vi "Dashboard Main.vi"() -> ()   [LabVIEW 2016]
uses:
  Auton Selector.ctl
  The-One-True-Robot-2017/Control Type.ctl
  <vilib>/Utility/miscctls.llb/LVRowAndColumnTypeDef.ctl
  <vilib>/event_ctls.llb/eventvkey.ctl
  <vilib>/Rock Robotics/Network Tables/NT Read Numeric Array.vi
  <vilib>/Rock Robotics/WPI/Dashboard/WPI_DashboardLogging Global.vi
  <vilib>/Rock Robotics/Network Tables/NT Write Boolean.vi
  <vilib>/Rock Robotics/Network Tables/NT Write Numeric Array.vi
  <vilib>/Rock Robotics/Network Tables/NT Write String Array.vi
panel:
  in  "Camera Settings Right":T1={"Frame Rate"=30, "Compression"=30, "Size"=1, "DB Camera Config"=FALSE} {"Frame Rate" scale=1.0..30.0; "Compression" scale=100.0..-1.0; "Size" items=["640x480", "320x240", "160x120"]}
  in  "Camera Name Right":string(combo)="No Camera Selection"
  out "Camera Info":cluster{"Mbps LED":bool, "Mbps":dbl, "fps":dbl} {"fps" format="%#.1g"; "Mbps" format="%#.1g"}
  in  "Camera Settings":T1={"Frame Rate"=30, "Compression"=30, "Size"=1, "DB Camera Config"=FALSE} {"Frame Rate" scale=1.0..30.0; "Compression" scale=100.0..-1.0; "Size" items=["640x480", "320x240", "160x120"]}
  in  "TCP":refnum<k5>
  in  "Rec Mode":enum32{"Stop", "Record", "Playback"}(radio)
  out "Robot IP":string
  out "Image Message":string="Timeout in Camera Communications"
  in  "Dashboard Tab":T2(tab)
  in  "Select Auto":T3="Select Autonomous ..."
  out "NT Connection":bool
  out "MotorChart R":cluster{"Numeric":dbl, "Numeric":dbl}(graph)
  out "MotorChart L":cluster{"Numeric":dbl, "Numeric":dbl}(graph)
  out "MotorSliders R":cluster{"MotorSlide1":dbl, "MotorSlide2":dbl} {"MotorSlide2" scale=-1.0..1.0 scale format="%#_2e"; "MotorSlide1" scale=-1.0..1.0 scale format="%#_2e"}
  out "MotorSliders L":cluster{"MotorSlide1":dbl, "MotorSlide2":dbl} {"MotorSlide2" scale=-1.0..1.0 scale format="%#_2e"; "MotorSlide1" scale=-1.0..1.0 scale format="%#_2e"}
  out "Gyro":dbl(knob) scale=0.0..360.0
  out "JS1 Z":dbl(slide) scale=-1.0..1.0 scale format="%#_2e"
  out "JS1 Graph":cluster{"X":dbl, "Y":dbl}[](graph)
  out "JS1 Buttons":T4
  out "JS2 Z":dbl(slide) scale=-1.0..1.0 scale format="%#_2e"
  out "JS2 Graph":cluster{"X":dbl, "Y":dbl}[](graph)
  out "JS2 Buttons":T4
  out "Mode":T5(ring)=enum."Auto Disabled"
  in  "Select Auto 3":T6
  out "Camera Image Right":T7(plugin-control)
  in  "DB/String 9":string
  in  "DB/String 8":string
  in  "DB/String 7":string
  in  "DB/String 6":string
  in  "DB/String 5":string
  in  "DB/String 4":string
  in  "DB/String 3":string
  in  "DB/String 2":string
  in  "DB/String 1":string
  in  "DB/String 0":string
  in  "DB/Slider 0":dbl(slide) scale=0.0..5.0
  in  "DB/Slider 1":dbl(slide) scale=0.0..5.0
  in  "DB/Slider 2":dbl(slide) scale=0.0..5.0
  in  "DB/Slider 3":dbl(slide) scale=0.0..5.0
  out "DB/LED 3":bool
  out "DB/LED 2":bool
  in  "DB/Button 3":bool
  in  "DB/Button 2":bool
  in  "DB/Button 1":bool
  in  "DB/Button 0":bool
  out "DB/LED 0":bool
  out "DB/LED 1":bool
  in  "Nintendo Camera Switch":bool
  in  "Distance":dbl
  in  "Right":dbl
  in  "Left":dbl
  in  "Toggle LED":bool
  in  "Test Slider":dbl(slide) scale=0.0..100.0 scale format="%#_3g"
  in  "On/Off":bool caption="Solenoid"
  in  "Test Name":u16(ring) items=["Select the test to run..."]
  in  "Test Tree":string(tree)
  in  "Motor":cluster{"Value":dbl, "Enable":bool} {"Value" scale=-1.0..1.0 scale format="%#_3g"}
  out "Progress":T8 {"Test Progress" scale=0.0..100.0}
  in  "Rev/Fwd":cluster{"Forward":bool, "Reverse":bool}
  in  "Test Ring":u16(ring) items=["Monochrome", "Color"]
  out "Cmd Status":string
  in  "Execute Command":bool
  in  "Command Params":string[][](table)
  in  "Command Selection":i32(listbox)
  in  "CheckList":i32(listbox)
  out "Tree":string(tree)
  out "Camera Image":T7(plugin-control)
  out "Background":bool
  in  "Camera Name":string(combo)="No Camera Selection"
  # "HW"
  # "HW"
  # "Joysticks"
  # "Drive Motors"
  # "Front"
  # "Right"
  # "Left"
  # "Back"
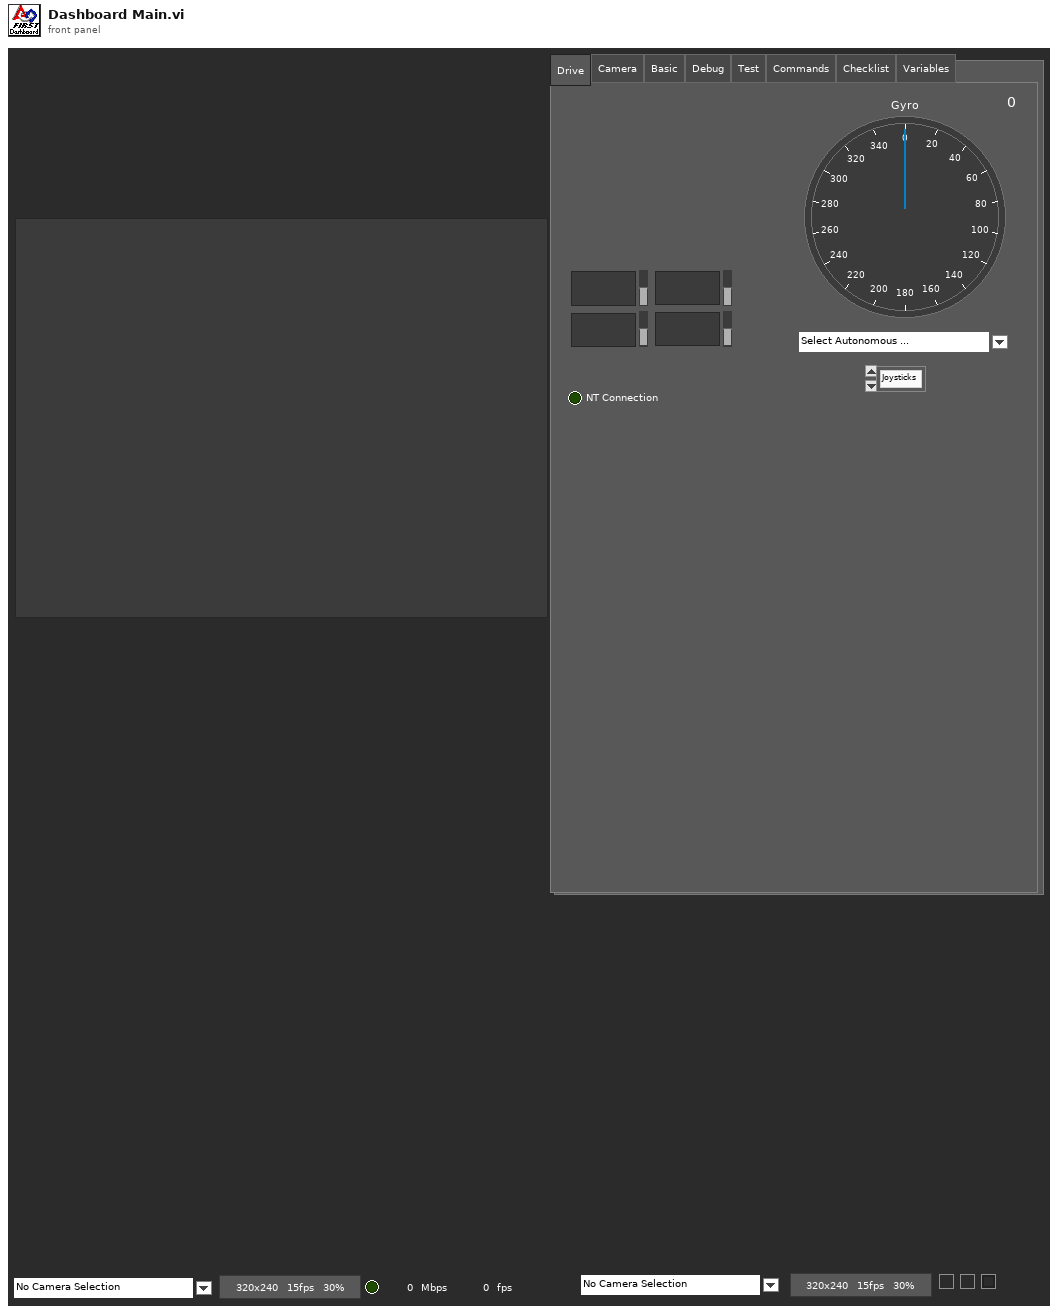
[diagram p1: front panel]
types:
  T1 = cluster{"Frame Rate":i32, "Compression":i32, "Size":u16, "DB Camera Config":bool}
  T2 = enum32{"Drive", "Camera", "Basic", "Debug", "Test", "Commands", "Checklist", "Variables"}
  T3 = typedef "Auton Selector.ctl" = string
  T4 = cluster{bool, bool, bool, bool, bool, bool, bool, bool, bool, bool, bool, bool}
  T5 = enum8{"Tele-Op Disabled", "Tele-Op Enabled", "Auto Disabled", "Auto Enabled", "Test Disabled", "Test Enabled", "Disconnected", "No Code", "E-Stop"}
  T6 = typedef "Control Type.ctl" = enum16{"Joysticks", "Xbox", "DancingRevolution"}
  T7 = typedef "IMAQ Image.ctl" = refnum<image>
  T8 = cluster{"Test Progress":u8, "Test Progress Text":string}
  T9 = typedef "Image Type" = u32
  T10 = cluster{"IDs":cluster{"RPC field ID":u16, "Unique ID":u16}, "String":string}
  T11 = enum32{"Drive", "Basic", "Debug", "Test", "Checklist", "Variables"}
  T12 = cluster{"Error Strings":string, "Disable Counts":cluster{u16, u16}, "Rail Faults":cluster{u16, u16, u16}, "Robot IP":string, "DB Mode":u8, "Event Info":cluster{"Name":string, "Type":u8, "Number":u16, "Replay":u8}}
  T13 = cluster{"Storage":cluster{"Disk Free":u64, "RAM Block":u32, "RAM free":u32}, "CPU Utilization":cluster{"CPU % ISR":sgl, "CPU % Time Crit":sgl, "CPU % Timed Str":sgl, "CPU % High":sgl, "CPU % Above":sgl, "CPU % Normal":sgl, "CPU % Low":sgl}, "CAN":cluster{"% Bus Utilization":sgl, "Bus Off Cnt":u32, "TX_FIFO Full Cnt":u32, "Receive Error Cnt":u8, "Transmit Error Cnt":u8}, "HID":cluster{"HID Outputs":u32, "Rumble Low":u16, "Rumble High":u16}[]}
  T14 = cluster{"Status bits":cluster{"Test Mode":bool, "Autonomous":bool, "Enabled":bool, "Code Start":bool, "Brownout":bool, "Reserved 2":bool, "Reserved 3":bool, "E-Stop":bool}, "Code Trace":cluster{"Disabled":bool, "TeleOp":bool, "Auto":bool, "Test":bool}, "Controller Type":enum16{"unknown", "cRIO", "roboRio"}, "Code?":enum16{"unknown", "noCode", "code"}, "Battery V":dbl}
  T15 = cluster{"Control Bits":cluster{"TestMode":bool, "Autonomous":bool, "Enabled":bool, "FMS Present":bool, bool, bool, bool, "E-Stop":bool}, "Team Station ":u8, "Countdown":sgl, "Joystick Values":cluster{"Axes":dbl[], "Buttons":bool[], "POVs":i16[]}[]}
  T16 = cluster{"Axes":dbl[], "Buttons":bool[], "POVs":i16[]}[]
  T17 = cluster{"Axes":dbl[], "Buttons":bool[], "POVs":i16[]}
  T18 = cluster{"Buttons[0]":bool, "Buttons[1]":bool, "Buttons[2]":bool, "Buttons[3]":bool, "Buttons[4]":bool, "Buttons[5]":bool, "Buttons[6]":bool, "Buttons[7]":bool, "Buttons[8]":bool, "Buttons[9]":bool, "Buttons[10]":bool, "Buttons[11]":bool}
  T19 = cluster{"Camera Image":refnum<vi>, "Dashboard Tab":refnum<vi>, "Background":refnum<vi>, "Rec Mode":refnum<vi>, "Test Slider":refnum<vi>, "On/Off ":refnum<vi>, "Test Ring":refnum<vi>, "Rev/Fwd":refnum<vi>, "Test Name":refnum<vi>, "Motor":refnum<vi>, "Progress":refnum<vi>, "CheckList":refnum<vi>, "Tree":refnum<vi>, "Test Tree":refnum<vi>, "Command Params":refnum<vi>, "Command Selection":refnum<vi>, "Execute Command":refnum<vi>, "Cmd Status":refnum<vi>, "Camera Settings":refnum<vi>, "Camera Name":refnum<vi>, "Camera Info":refnum<vi>, "Camera Settings Right":refnum<vi>, "Camera Name Right":refnum<vi>, "Camera Image Right":refnum<vi>}
  T20 = cluster{"Operation":enum16{"Update", "Clear"}, "Color Box":u32}[]
  T21 = typedef "eventvkey.ctl" = enum16{"ASCII", "Enter", "Return", "Shift", "Ctrl", "Alt", "Cmd", "Opt", "Caps", "NumLock", "Clear", "Break", "Up", "Down", "Left", "Right", "Insert", "Delete", "Home", "End", "PageUp", "PageDown", "Escape", "Help", "Pause", "ScrollLock", "F1", "F2", "F3", "F4", "F5", "F6", "F7", "F8", "F9", "F10", "F11", "F12", "F13", "F14", "F15", "F16", "F17", "F18", "F19", "F20", "F21", "F22", "F23", "F24", "Play", "VolumeUp", "VolumeDown", "Mute", "Two Byte Char"}
  T22 = cluster{"Image Size":bool, "Image Type":bool, "Pixel Value":bool, "ROI Information":bool, "Zoom Factor":bool}
  T23 = cluster{"Operation":enum16{"Update", "Clear"}, "Color Box":u32}
  T24 = typedef "LVRowAndColumnTypeDef.ctl" = cluster{"Row":i32, "Column":i32}
  T25 = cluster{"Shift":bool, "Ctrl":bool, "Alt":bool, "Cmd":bool, "Opt":bool}
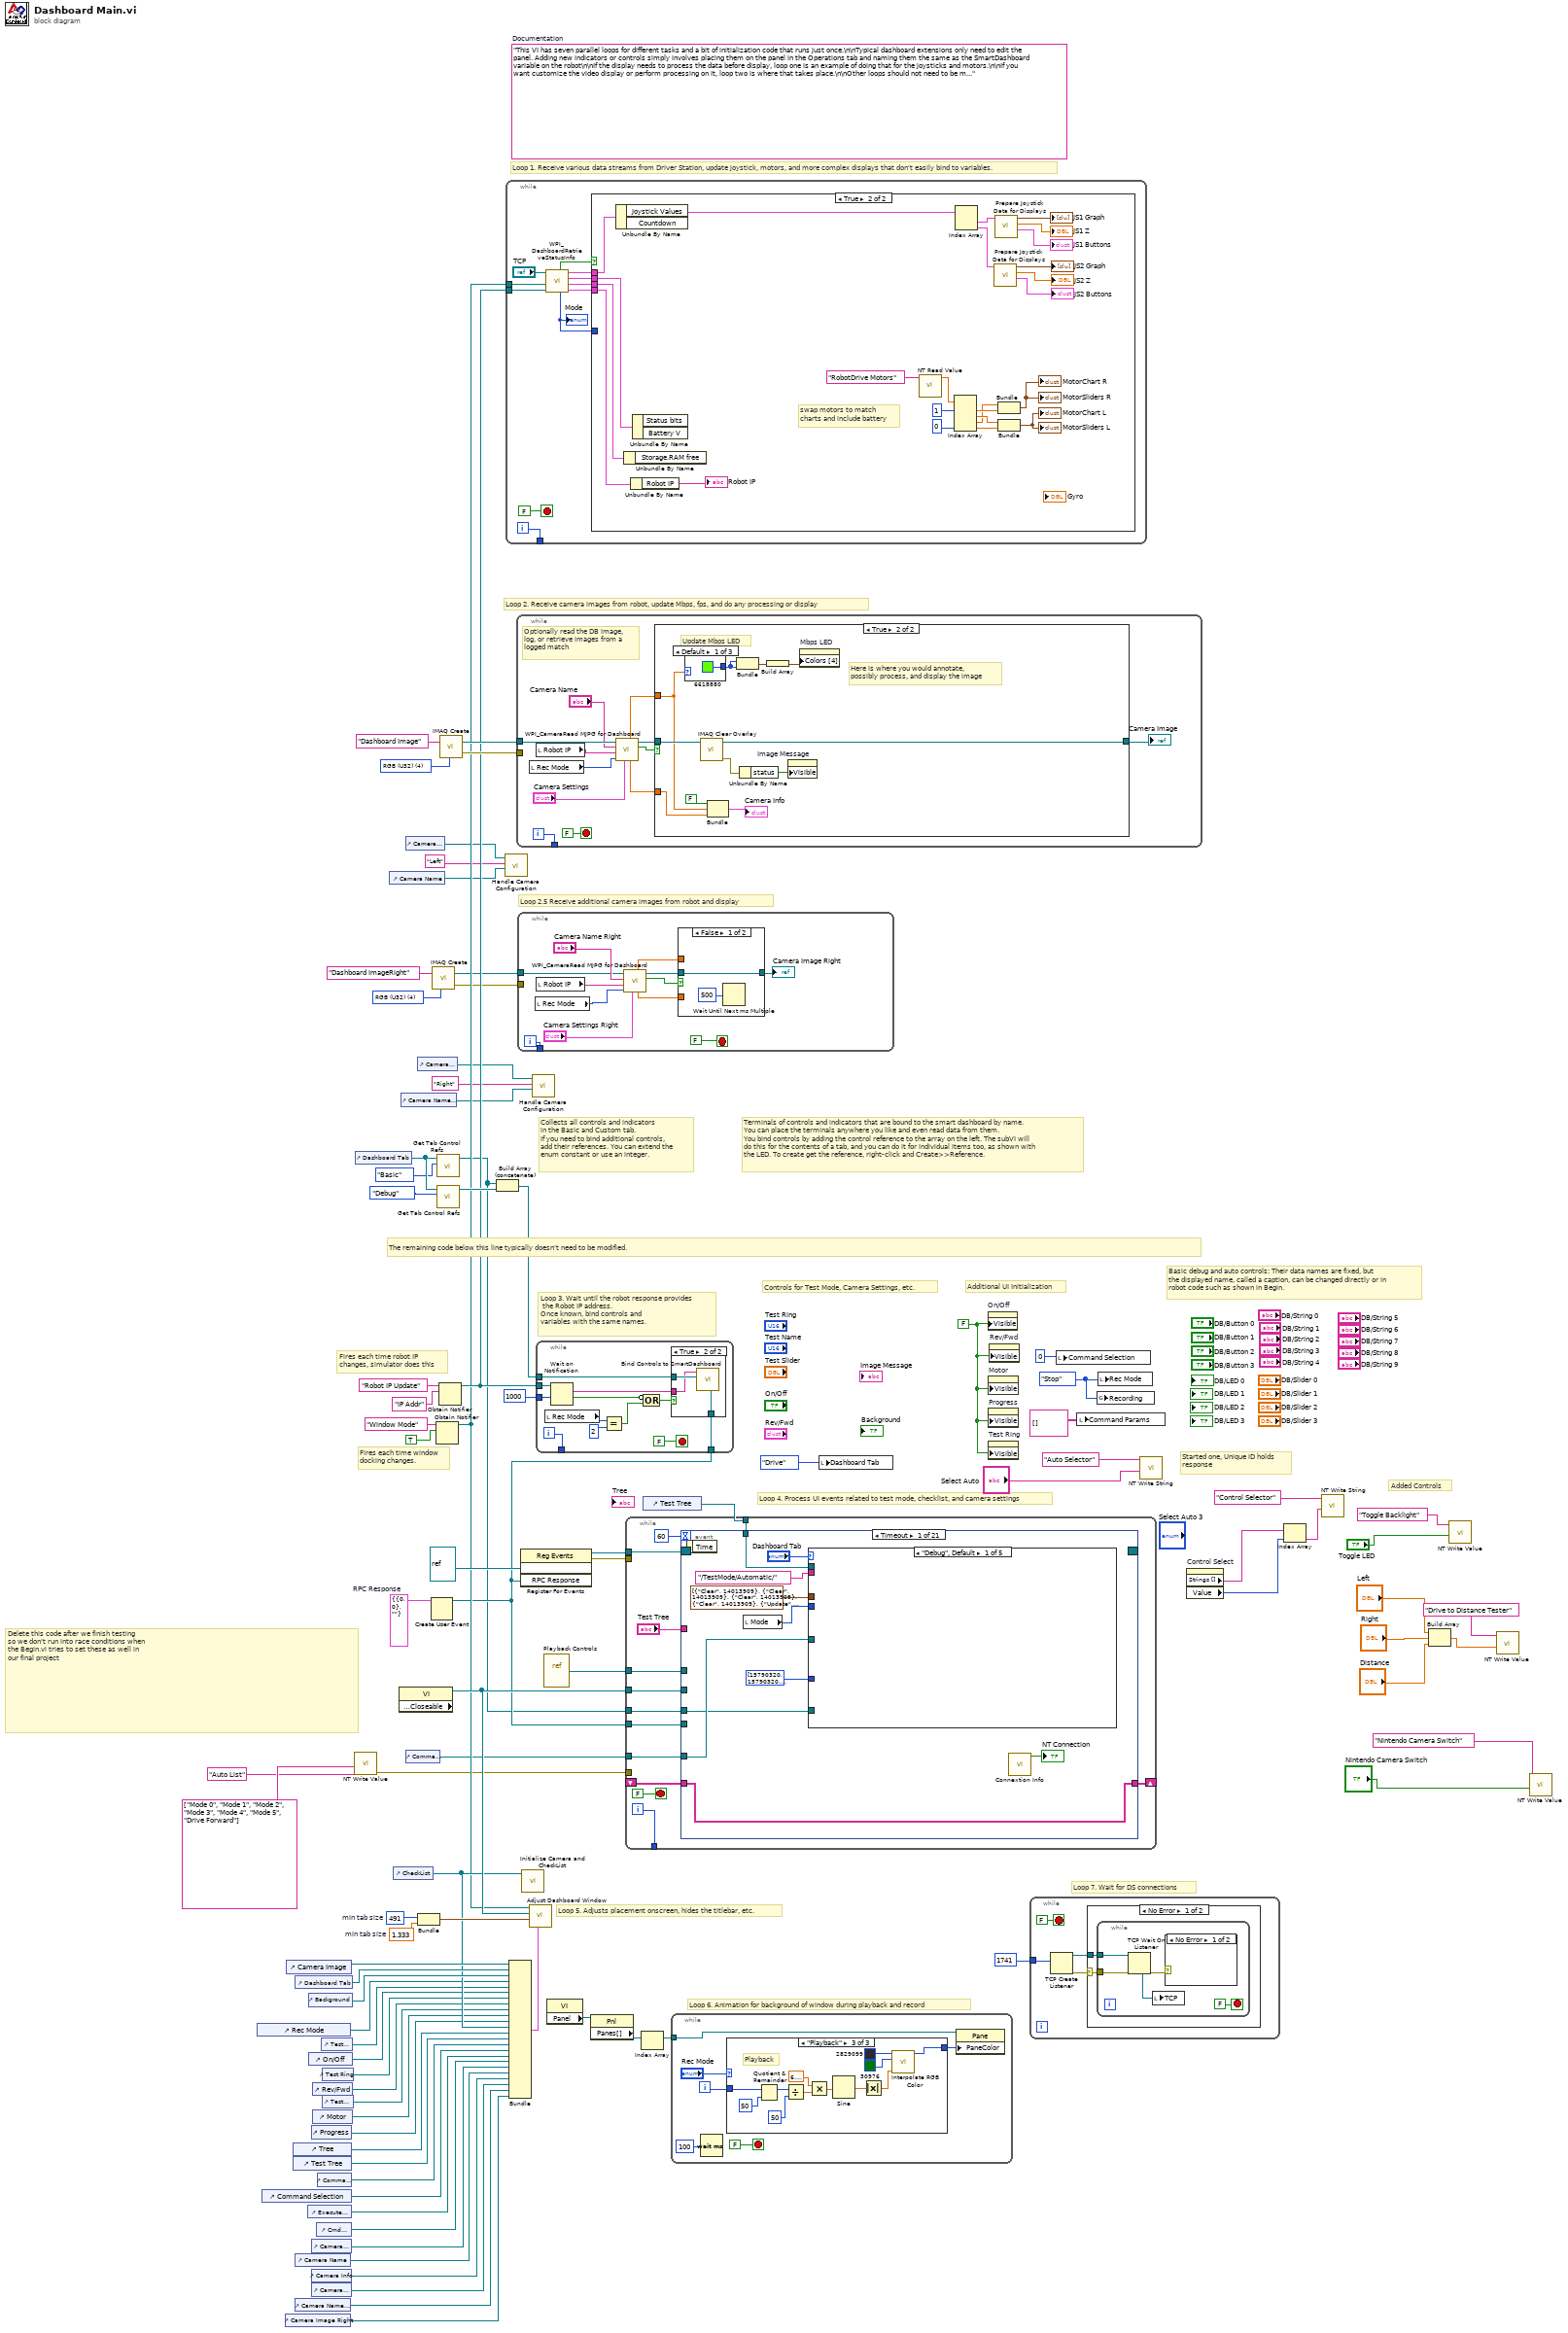
[diagram p0: block diagram]
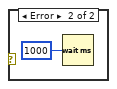
[diagram p3: hidden frame]
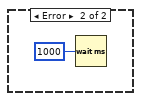
[diagram p4: hidden frame]
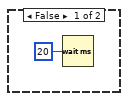
[diagram p5: hidden frame]
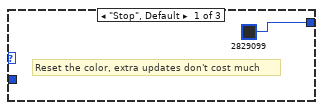
[diagram p6: hidden frame]
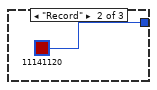
[diagram p7: hidden frame]
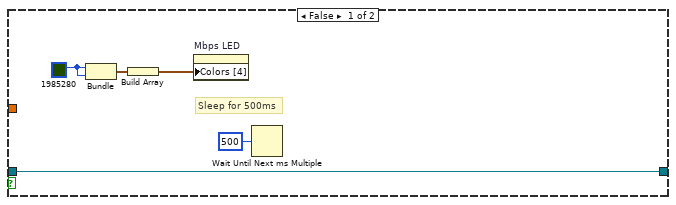
[diagram p9: hidden frame]
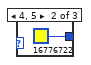
[diagram p10: hidden frame]
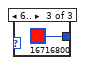
[diagram p11: hidden frame]
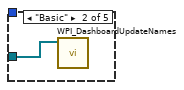
[diagram p12: hidden frame]
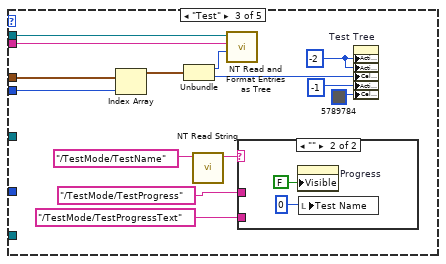
[diagram p13: hidden frame]
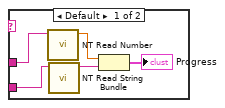
[diagram p14: hidden frame]
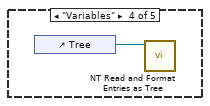
[diagram p15: hidden frame]
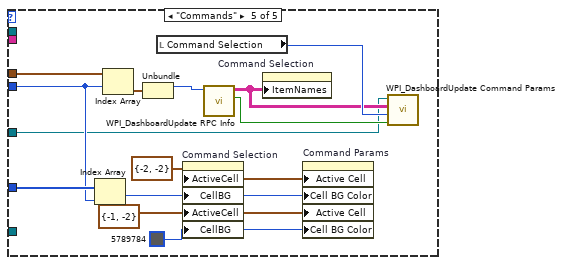
[diagram p16: hidden frame]
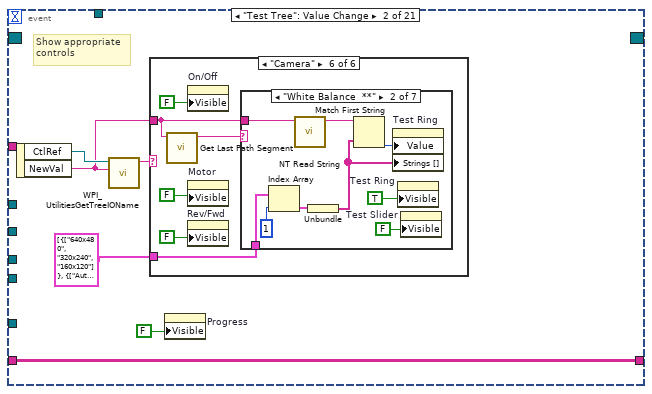
[diagram p17: hidden frame]
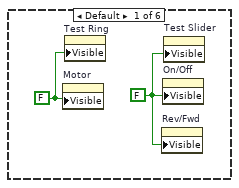
[diagram p18: hidden frame]
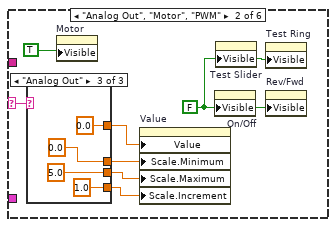
[diagram p19: hidden frame]
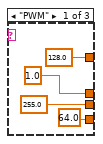
[diagram p20: hidden frame]
diagram:
  w27 = T9 4 items=["Grayscale (U8)", "Grayscale (I16)", "Grayscale (SGL)", "Complex (CSG)", "RGB (U32)", "HSL (U32)", "RGB (U64)"] ("Image Type")
  w42 = T10 {"IDs"={"RPC field ID"=0, "Unique ID"=0}, "String"=""}  # RPC Response
  w67 = 491  # min tab size
  w66 = 1.333  # min tab size
  w74 = enum32{"Stop", "Record", "Playback"}."Stop" ("Rec Mode")
  w49 = FALSE ("Visible")
  (unwired) "This VI has seven parallel loops for different tasks and a bit of initialization code that runs just once.\n\nTypical dashboard extensions only need to edit the panel. Adding new indicators or controls simply involves placing them on the panel in the Operations tab and naming them the same as the SmartDashboard variable on the robot\n\nIf the display needs to process the data before display, loop one is an example of doing that for the joysticks and motors.\n\nIf you want customize the video display or perform processing on it, loop two is where that takes place.\n\nOther loops should not need to be modified. They are pretty standard, and document the task they perform."  # Documentation
  w91 = T9 4 items=["Grayscale (U8)", "Grayscale (I16)", "Grayscale (SGL)", "Complex (CSG)", "RGB (U32)", "HSL (U32)", "RGB (U64)"] ("Image Type")
  # "Delete this code after we finish testing\nso we don't run into race conditions when\nthe Begin.vi tries to set these as well in\nour final project"
  # "Added Controls"
  # "Loop 2.5 Receive additional camera images from robot and display"
  # "Started one, Unique ID holds\nresponse"
  # "Loop 7. Wait for DS connections"
  # "Basic debug and auto controls: Their data names are fixed, but\nthe displayed name, called a caption, can be changed directly or in\nrobot code such as shown in Begin."
  # "Controls for Test Mode, Camera Settings, etc."
  # "Additional UI Initialization"
  # "Loop 6. Animation for background of window during playback and record"
  # "Fires each time robot IP\nchanges, simulator does this"
  # "Fires each time window\ndocking changes."
  # "Collects all controls and indicators\nin the Basic and Custom tab.\nIf you need to bind additional controls,\nadd their references. You can extend the\nenum constant or use an integer."
  # "The remaining code below this line typically doesn't need to be modified."
  # "Loop 4. Process UI events related to test mode, checklist, and camera settings"
  # "Terminals of controls and indicators that are bound to the smart dashboard by name.\nYou can place the terminals anywhere you like and even read data from them.\nYou bind controls by adding the control reference to the array on the left. The subVI will\ndo this for the contents of a tab, and you can do it for individual items too, as shown with\nthe LED. To create get the reference, right-click and Create>>Reference."
  # "Loop 3. Wait until the robot response provides\n the Robot IP address.\nOnce known, bind controls and\nvariables with the same names."
  # "Loop 5. Adjusts placement onscreen, hides the titlebar, etc."
  # "Loop 1. Receive various data streams from Driver Station, update joystick, motors, and more complex displays that don't easily bind to variables."
  # "Loop 2. Receive camera images from robot, update Mbps, fps, and do any processing or display"
  n1 = control-ref of="Rec Mode"() -> (w55:refnum<vi>)
  n2 = control-ref of="Command Selection"() -> (w41:refnum<vi>)
  n3 = control-ref of="Camera Image Right"() -> (w18:refnum<vi>)
  n4 = control-ref of="Camera Image"() -> (w69:refnum<vi>)
  n5 = control-ref of="Tree"() -> (w59:refnum<vi>)
  n6 = control-ref of="Test Tree"() -> (w58:refnum<vi>)
  n7 = control-ref of="Dashboard Tab"() -> (w68:refnum<vi>)
  n8 = control-ref of="Camera Name"() -> (w32:refnum<vi>)
  n9 = control-ref of="Camera Name Right"() -> (w19:refnum<vi>)
  n10 = control-ref of="Execute Command"() -> (w43:refnum<vi>)
  n11 = control-ref of="Background"() -> (w64:refnum<vi>)
  n12 = control-ref of="On/Off"() -> (w53:refnum<vi>)
  n13 = control-ref of="Progress"() -> (w50:refnum<vi>)
  n14 = control-ref of="Camera Settings"() -> (w33:refnum<vi>)
  n15 = control-ref of="Camera Info"() -> (w31:refnum<vi>)
  n16 = control-ref of="Camera Settings Right"() -> (w20:refnum<vi>)
  n17 = control-ref of="Rev/Fwd"() -> (w51:refnum<vi>)
  n18 = control-ref of="Motor"() -> (w56:refnum<vi>)
  n19 = control-ref of="Cmd Status"() -> (w37:refnum<vi>)
  n20 = control-ref of="Command Params"() -> (w44:refnum<vi>)
  n21 = control-ref of="Test Slider"() -> (w54:refnum<vi>)
  n22 = control-ref of="Test Ring"() -> (w52:refnum<vi>)
  n23 = control-ref of="Test Name"() -> (w57:refnum<vi>)
  n24 = call-poly <vilib>:"NT Write Value.vi"("String Array"=string[] ["Mode 0", "Mode 1", "Mode 2", "Mode 3", "Mode 4", "Mode 5", "Drive Forward"], "Name"="Auto List") -> ("error out"=w8:errorcluster)  [unwired: 9 in]
  n25 = control-ref of="Dashboard Tab"() -> (w72:refnum<vi>)
  n26 = control-ref of="Camera Name"() -> (w34:refnum<vi>)
  n27 = control-ref of="CheckList"() -> (w60:refnum<vi>)
  n28 = property class="VI" props=["Front Panel.Closeable"]() -> (reference out=w73:refnum<vi>)  [unwired: 2 in, 2 out]
  n29 = control-ref of="Camera Name Right"() -> (w23:refnum<vi>)
  n30 = control-ref of="Camera Settings"() -> (w35:refnum<vi>)
  n31 = control-ref of="Command Params"() -> (w36:refnum<vi>)
  n32 = control-ref of="Camera Settings Right"() -> (w24:refnum<vi>)
  n33 = Bundle("min tab size"=w67, "min tab size"=w66) -> (w65:cluster{"min tab size":i32, "min tab size":dbl})  [unwired: 1 in]
  n34 = Create User Event(user event datatype=w42) -> (user event=w38:refnum<user-event>)  [unwired: 1 in, 1 out]
  n35 = call "IMAQ Create"("Image Name"="Dashboard ImageRight", "Image Type"=w27) -> ("New Image"=w26:T7, "error out"=w25:errorcluster)  [unwired: 2 in, 1 out]
  n36 = Obtain Notifier(name (unnamed)="Window Mode", notification data type=TRUE) -> (notifier out=w47:refnum<notifier>)  [unwired: 2 in, 2 out]
  n37 = call <vilib>:"Get Tab Control Refs.vi"("Page Index"=T11."Basic" ("Dashboard Tab"), "TabControl in"=w72) -> ("ControlsOnPage"=w30:refnum<vi>[])  [unwired: 9 in]
  n38 = call <vilib>:"Get Tab Control Refs.vi"("Page Index"=T11."Debug" ("Dashboard Tab"), "TabControl in"=w72) -> ("ControlsOnPage"=w71:refnum<vi>[])  [unwired: 9 in]
  n39 = Obtain Notifier(name (unnamed)="Robot IP Update", notification data type="IP Addr" ("name (unnamed)")) -> (notifier out=w48:refnum<notifier>)  [unwired: 2 in, 2 out]
  n40 = call "IMAQ Create"("Image Name"="Dashboard Image", "Image Type"=w91) -> ("New Image"=w89:T7, "error out"=w88:errorcluster)  [unwired: 2 in, 1 out]
  n41 = Build Array (concatenate)(w30, w71) -> (w70:refnum<vi>[])
  n42 = call "Handle Camera Configuration.vi"("CameraNameRef"=w34, "Camera File Name"="Left", "ClusterRef"=w35) -> ()  [unwired: 9 in]
  n43 = while {
    tunnel: [w101] -> _
    tunnel: w48 -> [w95]
    tunnel: w47 -> [w92]
    i -> [w101]
    stop <- FALSE stop-if-true
    n44 = call <vilib>:"WPI_DashboardRetrieveStatusInfo.vi"("Binding Refnum"=w95, "Window Mode Notifier"=w92, "TCP Cnx"="TCP") -> ("Power and Errors"=w96:T12, "Robot Metrics"=w99:T13, "Status Info"=w100:T14, "Control Info"=w97:T15, "Robot Mode"=w94:T5, "Process?"=w98:bool)  [unwired: 3 in]
    "Mode" <- w94
    n45 = case shown="True" w98 {
      tunnel: w100 -> [_ w127]
      tunnel: w99 -> [_ w126]
      tunnel: w97 -> [_ w125]
      tunnel: w96 -> [_ w124]
      tunnel: w94 -> [_ _]
      frame False {
        n46 = Wait (ms)(milliseconds to wait=u32 20) -> ()  [unwired: 1 out]
      }
      frame True {
        # "swap motors to match\ncharts and include battery"
        n47 = Unbundle By Name(w125) -> ("Joystick Values"=w115:T16)  [unwired: 1 out]
        n48 = Unbundle By Name(w126) -> ()  [unwired: 1 out]
        n49 = Unbundle By Name(w124) -> ("Robot IP"=→"Robot IP":string)
        n50 = Unbundle By Name(w127) -> ()  [unwired: 2 out]
        n51 = call-poly <vilib>:"NT Read Value.vi"("Name"="RobotDrive Motors") -> ("Numeric Array"=w105:dbl[])  [unwired: 9 in, 1 out]
        n52 = Index Array(array=w105, index #1=1, index #4=0) -> (element #1=w119:dbl, element #2=w120:dbl, element #3=w118:dbl, element #4=w123:dbl)  [unwired: 2 in]
        n53 = Index Array(array=w115) -> (element #1=w114:T17, element #2=w110:T17)  [unwired: 2 in]
        n54 = call "Prepare Joystick Data for Displays.vi"("Joystick Values"=w110) -> ("Buttons"=→"JS2 Buttons":T18, "Z Axis"=→"JS2 Z":dbl, "Cartesian Data"=→"JS2 Graph":cluster{"X axis":dbl, "X axis":dbl}[])  [unwired: 8 in]
        n55 = call "Prepare Joystick Data for Displays.vi"("Joystick Values"=w114) -> ("Buttons"=→"JS1 Buttons":T18, "Z Axis"=→"JS1 Z":dbl, "Cartesian Data"=→"JS1 Graph":cluster{"X axis":dbl, "X axis":dbl}[])  [unwired: 8 in]
        n56 = Bundle("Numeric"=w118, "Numeric"=w119) -> (→"MotorChart R" →"MotorSliders R":cluster{"Numeric":dbl, "Numeric":dbl})  [unwired: 1 in]
        n57 = Bundle("Numeric"=w120, "Numeric"=w123) -> (→"MotorChart L" →"MotorSliders L":cluster{"Numeric":dbl, "Numeric":dbl})  [unwired: 1 in]
      }
    }
  }
  n58 = Bundle("Camera Image"=w69, "Dashboard Tab"=w68, "Background"=w64, "Rec Mode"=w55, "Test Slider"=w54, "On/Off"=w53, "Test Ring"=w52, "Rev/Fwd"=w51, "Test Name"=w57, "Motor"=w56, "Progress"=w50, "CheckList"=w60, "Tree"=w59, "Test Tree"=w58, "Command Params"=w44, "Command Selection"=w41, "Execute Command"=w43, "Cmd Status"=w37, "Camera Settings"=w33, "Camera Name"=w32, "Camera Info"=w31, "Camera Settings Right"=w20, "Camera Name Right"=w19, "Camera Image Right"=w18) -> (w61:T19)  [unwired: 1 in]
  n59 = while {
    tunnel: w89 -> [w137]
    tunnel: w88 -> [_]
    tunnel: [w138] -> _
    i -> [w138]
    stop <- FALSE stop-if-true
    # "Optionally read the DB image,\nlog, or retrieve images from a\nlogged match"
    n60 = local read "Rec Mode"() -> (w133:enum32{"Stop", "Record", "Playback"})
    n61 = local read "Robot IP"() -> (w132:string)
    n62 = call <vilib>:"WPI_CameraRead MJPG for Dashboard.vi"("Camera Settings"="Camera Settings", "Rec Mode"=w133, "Robot IP"=w132, "Camera Name"="Camera Name", "Refnum in"=w137) -> ("Active"=w135:bool, "Refnum out"=w136:T7, "FPS"=w134:dbl, "Bandwidth (Mbps)"=w131:dbl)  [unwired: 3 in]
    n63 = case shown="True" w135 {
      tunnel: w136 -> [w140 w151]
      tunnel: w131 -> [_ w148]
      tunnel: w134 -> [_ w149]
      tunnel: [w140 w145] -> w128
      frame False {
        w142 = u32 1985280 ("Color Box")
        # "Sleep for 500ms"
        n64 = Bundle("Color Box"=w142, "Color Box"=w142) -> (w143:cluster{"Color Box":u32, "Color Box":u32})  [unwired: 1 out]
        n65 = Build Array(w143) -> (w141:cluster{"Color Box":u32, "Color Box":u32}[])
        n66 = property on="Mbps LED" class="Bool (strict)"("Colors [4]"=w141) -> ()  [unwired: 2 in, 2 out]
        n67 = Wait Until Next ms Multiple(millisecond multiple=u32 500) -> ()  [unwired: 1 out]
      }
      frame True {
        # "Here is where you would annotate,\npossibly process, and display the image"
        # "Update Mbps LED"
        n68 = case shown="Default" w148 {
          tunnel: [u32 6618880 ("Color Box") u32 16776722 ("Color Box") u32 16716800 ("Color Box")] -> w152
          frame Default {
          }
          frame 4, 5 {
          }
          frame 6.. {
          }
        }
        n69 = call "IMAQ Clear Overlay"("Image"=w151) -> ("error out"=w154:errorcluster, "Image Out"=w145:T7)  [unwired: 2 in, 7 out]
        n70 = Bundle(FALSE, "Bandwidth (Mbps)"=w148, "FPS"=w149) -> (→"Camera Info":cluster{bool, "Bandwidth (Mbps)":dbl, "FPS":dbl})  [unwired: 1 in]
        n71 = Bundle("Color Box"=w152, "Color Box"=w152) -> (w153:cluster{"Color Box":u32, "Color Box":u32})  [unwired: 1 out]
        n72 = Unbundle By Name(w154) -> ("status"=w155:bool)
        n73 = Build Array(w153) -> (w150:cluster{"Color Box":u32, "Color Box":u32}[])
        n74 = property on="Image Message" class="Str"("Visible"=w155) -> ()  [unwired: 2 in, 2 out]
        n75 = property on="Mbps LED" class="Bool (strict)"("Colors [4]"=w150) -> ()  [unwired: 2 in, 2 out]
      }
    }
    "Camera Image" <- w128
  }
  n76 = while {
    tunnel: w26 -> [w169]
    tunnel: w25 -> [_]
    tunnel: [w163] -> _
    i -> [w163]
    stop <- FALSE stop-if-true
    n77 = local read "Rec Mode"() -> (w167:enum32{"Stop", "Record", "Playback"})
    n78 = local read "Robot IP"() -> (w168:string)
    n79 = call <vilib>:"WPI_CameraRead MJPG for Dashboard.vi"("Camera Settings"="Camera Settings Right", "Rec Mode"=w167, "Robot IP"=w168, "Camera Name"="Camera Name Right", "Refnum in"=w169) -> ("Active"=w162:bool, "Refnum out"=w165:T7, "FPS"=w160:dbl, "Bandwidth (Mbps)"=w161:dbl)  [unwired: 3 in]
    n80 = case shown="False" w162 {
      tunnel: w165 -> [w171 w173]
      tunnel: w161 -> [_ _]
      tunnel: w160 -> [_ _]
      tunnel: [w171 w173] -> w159
      frame False {
        n81 = Wait Until Next ms Multiple(millisecond multiple=u32 500) -> ()  [unwired: 1 out]
      }
      frame True {
      }
    }
    "Camera Image Right" <- w159
  }
  n82 = register-events(refnum<vi> refnum, w38) -> (reference out=w78:refnum<event-registration>, error out=w77:errorcluster)  [unwired: 2 in]
  n83 = call "Initialize Camera and CheckList.vi"("ListBox in"=w60) -> ()  [unwired: 11 in]
  n84 = call "Adjust Dashboard Window.vi"("Sizing Refnums"=w61, "Size Constraints"=w65, "VI"=w73, "WIn Mode"=w47) -> ()  [unwired: 8 in]
  n85 = call "Handle Camera Configuration.vi"("CameraNameRef"=w23, "Camera File Name"="Right", "ClusterRef"=w24) -> ()  [unwired: 9 in]
  n86 = while {
    tunnel: w70 -> [w185]
    tunnel: w48 -> [w183]
    tunnel: [w181] -> _
    tunnel: u32 1000 ("milliseconds to wait") -> [w180]
    tunnel: w38 -> [w174]
    i -> [w181]
    stop <- FALSE stop-if-true
    n87 = local read "Rec Mode"() -> (w176:enum32{"Stop", "Record", "Playback"})
    n88 = Wait on Notification(notifier=w183, timeout in ms (-1)=w180) -> (notification=w182:string, timed out?=w178:bool)  [unwired: 2 in, 2 out]
    n89 = Equal?(x=w176, y=u16 2 ("Rec Mode")) -> (x = y?=w177:bool)
    n90 = Compound Arithmetic op=OR(invert w178, w177) -> (w179:bool)
    n91 = case shown="True" w179 {
      tunnel: w185 -> [_ w188]
      tunnel: w182 -> [_ w187]
      tunnel: w174 -> [_ w186]
      frame False {
      }
      frame True {
        n92 = call <vilib>:"Bind Controls to SmartDashboard.vi"("RPC ref"=w186, "Bound Control Refs"=w188, "Server IP Address"=w187) -> ()  [unwired: 9 in]
      }
    }
  }
  n93 = vi-ref "Playback Controls.vi"() -> (w79:refnum<vi>)
  n94 = property class="VI"() -> ("Panel"=w81:refnum<vi>)  [unwired: 2 in, 2 out]
  n95 = property class="Pnl"(reference=w81) -> ("Panes[]"=w82:refnum<vi>[])  [unwired: 1 in, 2 out]
  n96 = Index Array(array=w82) -> (element=w80:refnum<vi>)  [unwired: 1 in]
  n97 = control-ref of="Test Tree"() -> (w83:refnum<vi>)
  n98 = while {
    tunnel: [w198] -> _
    tunnel: w83 -> [w197]
    tunnel: w79 -> [w196]
    tunnel: w78 -> [w195]
    tunnel: w77 -> [_]
    tunnel: w73 -> [w194]
    tunnel: w38 -> [w193]
    tunnel: w36 -> [w192]
    shift-right: [w191] -> _
    shift-left: _ -> [w190]
    tunnel: w30 -> [w189]
    tunnel: w8 -> [_]
    i -> [w198]
    stop <- FALSE stop-if-true
    n99 = event shown="[0] Timeout" {
      selector: w195 -> [_ _ _ _ _ _ _ _ _ _ _ _ _ _ _ _ _ _ _ _ _]
      dyn-events: [_ _ _ _ _ _ _ _ _ _ _ _ _ _ _ _ w454 _ _ _ _] -> _
      timeout: u32 60 ("milliseconds to wait") -> [_ _ _ _ _ _ _ _ _ _ _ _ _ _ _ _ _ _ _ _ _]
      tunnel: w197 -> [w210 _ _ _ _ _ _ _ _ _ _ _ _ _ _ _ _ _ _ _ _]
      tunnel: "Test Tree" -> [_ _ _ _ _ _ _ _ _ _ _ w421 w429 w431 w435 w443 _ _ _ _ _]
      tunnel: w196 -> [_ _ _ _ _ _ _ _ _ _ _ _ _ _ _ _ w456 _ w474 _ _]
      tunnel: w194 -> [_ _ _ _ _ _ _ _ _ _ _ _ _ _ _ _ w452 _ _ _ _]
      tunnel: w193 -> [_ _ _ _ _ _ _ _ _ _ _ _ _ _ _ _ w448 _ _ _ _]
      tunnel: w192 -> [w205 _ _ _ _ _ w372 _ _ _ _ _ _ _ _ _ _ _ _ _ _]
      tunnel: [w204 w249 w351 w356 w365 w369 w370 w379 w389 w396 w408 w420 w427 w430 w434 w442 w447 w469 w471 w475 w486] -> w191
      tunnel: w190 -> [w204 w249 w351 w356 w365 w369 w370 _ _ w396 w408 w420 w427 w430 w434 w442 w447 w469 w471 w475 w486]
      tunnel: w189 -> [w202 _ _ _ _ _ _ _ _ _ _ _ _ _ _ _ _ _ _ _ _]
      event Timeout {
        n100 = event-data() -> ()  [unwired: 1 in, 1 out]
        n101 = local read "Mode"() -> (w207:T5)
        n102 = case shown="\"Debug\", Default" "Dashboard Tab" {
          tunnel: w210 -> [_ _ w226 _ _]
          tunnel: "/TestMode/Automatic/" ("Name Pattern") -> [_ _ w225 _ _]
          tunnel: T20 [{"Operation"=enum."Clear", "Color Box"=14013909}, {"Operation"=enum."Clear", "Color Box"=14013909}, {"Operation"=enum."Clear", "Color Box"=14013909}, {"Operation"=enum."Clear", "Color Box"=14013909}, {"Operation"=enum."Update", "Color Box"=14013909}, {"Operation"=enum."Update", "Color Box"=16777215}, {"Operation"=enum."Clear", "Color Box"=14013909}, {"Operation"=enum."Clear", "Color Box"=14013909}, {"Operation"=enum."Clear", "Color Box"=14013909}] -> [_ _ w218 _ w242]
          tunnel: w207 -> [_ _ w217 _ w241]
          tunnel: u32[] [15790320, 15790320, 15790320, 15790320, 16777215, 16777215, 15790320, 15790320, 15790320] -> [_ _ _ _ w247]
          tunnel: w205 -> [_ _ _ _ w235]
          tunnel: w202 -> [_ w212 _ _ _]
          frame "Debug", Default {
          }
          frame "Basic" {
            n103 = call <vilib>:"WPI_DashboardUpdateNames.vi"("Controls on Tab"=w212) -> ()  [unwired: 11 in]
          }
          frame "Test" {
            w224 = -2 ("Active Item:Row Number")
            n104 = Index Array(array=w218, index=w217) -> (element=w219:T23)
            n105 = Unbundle(w219) -> ("Operation"=w220:enum16{"Update", "Clear"}, "Color Box"=w221:u32)
            n106 = call <vilib>:"NT Read String.vi"("Name"="/TestMode/TestName") -> ("String"=w215:string)  [unwired: 9 in, 1 out]
            n107 = call <vilib>:"NT Read and Format Entries as Tree.vi"("Operation"=w220, "Name Pattern"=w225, "Tree Refnum"=w226) -> ()  [unwired: 7 in, 2 out]
            n108 = case shown="\"\"" w215 {
              tunnel: "/TestMode/TestProgress" ("Name") -> [w228 _]
              tunnel: "/TestMode/TestProgressText" ("Name") -> [w227 _]
              frame Default {
                n109 = call <vilib>:"NT Read Number.vi"("Name"=w228) -> ("Numeric"=w229:dbl)  [unwired: 9 in, 1 out]
                n110 = call <vilib>:"NT Read String.vi"("Name"=w227) -> ("String"=w230:string)  [unwired: 9 in, 1 out]
                n111 = Bundle("Numeric"=w229, "String"=w230) -> (→"Progress":cluster{"Numeric":dbl, "String":string})  [unwired: 1 in]
              }
              frame "" {
                n112 = property on="Progress" class="Clust (strict)"("Visible"=FALSE) -> ()  [unwired: 2 in, 2 out]
                n113 = local write "Test Name"(u16 0) -> ()
              }
            }
            n114 = property on="Test Tree" class="Tree (strict)"("Active Item Row Number"=w224, "ActiveColNum"=w224, "CellBG"=w221, "Active Item Row Number"=-1 ("Active Item:Row Number"), "CellBG"=u32 5789784 ("Color Box")) -> ()  [unwired: 2 in, 2 out]
          }
          frame "Variables" {
            n115 = control-ref of="Tree"() -> (w234:refnum<vi>)
            n116 = call <vilib>:"NT Read and Format Entries as Tree.vi"("Tree Refnum"=w234) -> ()  [unwired: 9 in, 2 out]
          }
          frame "Commands" {
            w243 = u32 5789784 ("Color Box")
            w244 = T24 {"Row"=-1, "Column"=-2} ("Active Cell:Active Cell")
            w246 = T24 {"Row"=-2, "Column"=-2} ("Active Cell:Active Cell")
            n117 = Index Array(array=w247, index=w241) -> (element=w245:u32)
            n118 = Index Array(array=w242, index=w241) -> (element=w240:T23)
            n119 = Unbundle(w240) -> ("Operation"=w239:enum16{"Update", "Clear"})  [unwired: 1 out]
            n120 = local read "Command Selection"() -> (w238:i32)
            n121 = property on="Command Selection" class="MCListbox (strict)"("ActiveCell"=w246, "CellBG"=w245, "ActiveCell"=w244, "CellBG"=w243) -> ()  [unwired: 2 in, 2 out]
            n122 = call <vilib>:"WPI_DashboardUpdate RPC Info.vi"("Operation"=w239) -> ("update"=w237:bool, "commands"=w236:string[][])  [unwired: 9 in]
            n123 = property on="Command Selection" class="MCListbox (strict)"("ItemNames"=w236) -> ()  [unwired: 2 in, 2 out]
            n124 = property on="Command Params" class="Tbl (strict)"("Active Cell"=w246, "Cell BG Color"=w245, "Active Cell"=w244, "Cell BG Color"=w243) -> ()  [unwired: 2 in, 2 out]
            n125 = call <vilib>:"WPI_DashboardUpdate Command Params.vi"("Update"=w237, "NewVal"=w238, "Commands"=w236, "Param Tbl"=w235) -> ()  [unwired: 7 in, 1 out]
          }
        }
        n126 = call <vilib>:"Connextion Info.vi"() -> ("Connected"=→"NT Connection":bool)  [unwired: 10 in, 1 out]
      }
      event "Test Tree": Value Change {
        # "Show appropriate\ncontrols"
        n127 = event-data() -> ("CtlRef"=w252:refnum<vi>, "NewVal"=w250:string)  [unwired: 1 in]
        n128 = call <vilib>:"WPI_UtilitiesGetTreeIOName.vi"("NewVal"=w250, "TreeControl in"=w252) -> ("I/O Name"=w253:string)  [unwired: 9 in]
        n129 = case shown="\"Camera\"" w253 {
          selector: w253 -> [_ w260 _ w282 w291 _]
          tunnel: w250 -> [_ _ w279 w281 _ w298]
          tunnel: cluster{string[]}[] [{["640x480", "320x240", "160x120"]}, {["Auto", "Fixed indoor", "Fixed outdoor 1", "Fixed outdoor 2", "Fixed fluorescent 1", "Fixed fluorescent 2", "Hold current"]}, {["Auto", "Flicker-free 50 Hz", "Flicker-free 60 Hz", "Hold current"]}, {["None", "Prioritize frame rate", "Prioritize image quality"]}, {["Monochrome", "Color"]}] -> [_ _ _ _ _ w297]
          frame Default {
            w255 = FALSE ("Visible")
            w254 = FALSE ("Visible")
            n130 = property on="Motor" class="Clust (strict)"("Visible"=w254) -> ()  [unwired: 2 in, 2 out]
            n131 = property on="Test Ring" class="Ring (strict)"("Visible"=w254) -> ()  [unwired: 2 in, 2 out]
            n132 = property on="Rev/Fwd" class="Clust (strict)"("Visible"=w255) -> ()  [unwired: 2 in, 2 out]
            n133 = property on="On/Off" class="Bool (strict)"("Visible"=w255) -> ()  [unwired: 2 in, 2 out]
            n134 = property on="Test Slider" class="Slide (strict)"("Visible"=w255) -> ()  [unwired: 2 in, 2 out]
          }
          frame "Analog Out", "Motor", "PWM" {
            w261 = FALSE ("Visible")
            n135 = case shown="\"Analog Out\"" w260 {
              tunnel: [1.0 ("Value") -1.0 ("Value") 0.0 ("Value")] -> w259
              tunnel: [255.0 ("Value") 1.0 ("Value") 5.0 ("Value")] -> w258
              tunnel: [128.0 ("Value") 0.0 ("Value") 0.0 ("Value")] -> w257
              tunnel: [64.0 ("Value") 0.5 ("Value") 1.0 ("Value")] -> w256
              frame "PWM" {
              }
              frame "Motor", Default {
              }
              frame "Analog Out" {
              }
            }
            n136 = property on="Motor" class="Clust (strict)"("Visible"=TRUE) -> ()  [unwired: 2 in, 2 out]
            n137 = property on="Value" class="Slide (strict)"("Value"=w257, "Scale.Minimum"=w259, "Scale.Maximum"=w258, "Scale.Increment"=w256) -> ()  [unwired: 2 in, 2 out]
            n138 = property on="On/Off" class="Bool (strict)"("Visible"=w261) -> ()  [unwired: 2 in, 2 out]
            n139 = property on="Test Slider" class="Slide (strict)"("Visible"=w261) -> ()  [unwired: 2 in, 2 out]
            n140 = property on="Test Ring" class="Ring (strict)"("Visible"=w261) -> ()  [unwired: 2 in, 2 out]
            n141 = property on="Rev/Fwd" class="Clust (strict)"("Visible"=w261) -> ()  [unwired: 2 in, 2 out]
          }
          frame "Servo" {
            w277 = FALSE ("Visible")
            n142 = call <vilib>:"NT Read Number.vi"("Name"=w279) -> ("Numeric"=w278:dbl)  [unwired: 9 in, 1 out]
            n143 = property on="Test Slider" class="Slide (strict)"("Visible"=TRUE, "Scale.Maximum"=170.0 ("Scale.Range:Maximum")) -> ()  [unwired: 2 in, 2 out]
            n144 = local write "Test Slider"(w278) -> ()
            n145 = property on="Motor" class="Clust (strict)"("Visible"=w277) -> ()  [unwired: 2 in, 2 out]
            n146 = property on="Rev/Fwd" class="Clust (strict)"("Visible"=w277) -> ()  [unwired: 2 in, 2 out]
            n147 = property on="On/Off" class="Bool (strict)"("Visible"=w277) -> ()  [unwired: 2 in, 2 out]
            n148 = property on="Test Ring" class="Ring (strict)"("Visible"=w277) -> ()  [unwired: 2 in, 2 out]
          }
          frame "Relay", "Solenoid" {
            w280 = FALSE ("Visible")
            n149 = property on="Motor" class="Clust (strict)"("Visible"=w280) -> ()  [unwired: 2 in, 2 out]
            n150 = property on="Test Slider" class="Slide (strict)"("Visible"=w280) -> ()  [unwired: 2 in, 2 out]
            n151 = Search and Replace String(input string=w281, search string="/Value  **", replace string="/Direction") -> (result string=w287:string)  [unwired: 5 in, 3 out]
            n152 = property on="Test Ring" class="Ring (strict)"("Visible"=w280) -> ()  [unwired: 2 in, 2 out]
            n153 = call <vilib>:"NT Read String.vi"("Name"=w287) -> ("String"=w285:string)  [unwired: 9 in, 1 out]
            n154 = Equal?(x="Both directions", y=w285) -> (x = y?=w283:bool)
            n155 = Not(x=w283) -> (.not. x?=w284:bool)
            n156 = property on="Rev/Fwd" class="Clust (strict)"("Visible"=w283) -> ()  [unwired: 2 in, 2 out]
            n157 = property on="On/Off" class="Bool (strict)"("Visible"=w284, "Caption.Text"=w282) -> ()  [unwired: 2 in, 2 out]
          }
          frame "Compressor", "Digital Out" {
            w290 = FALSE ("Visible")
            # "Get direction and finish"
            n158 = property on="Motor" class="Clust (strict)"("Visible"=w290) -> ()  [unwired: 2 in, 2 out]
            n159 = property on="Test Slider" class="Slide (strict)"("Visible"=w290) -> ()  [unwired: 2 in, 2 out]
            n160 = property on="Test Ring" class="Ring (strict)"("Visible"=w290) -> ()  [unwired: 2 in, 2 out]
            n161 = property on="On/Off" class="Bool (strict)"("Visible"=TRUE, "Caption.Text"=w291) -> ()  [unwired: 2 in, 2 out]
            n162 = property on="Rev/Fwd" class="Clust (strict)"("Visible"=FALSE) -> ()  [unwired: 2 in, 2 out]
          }
          frame "Camera" {
            n163 = call <vilib>:"Get Last Path Segment.vi"("String in"=w298) -> ("String out"=w299:string)  [unwired: 10 in]
            n164 = property on="On/Off" class="Bool (strict)"("Visible"=FALSE) -> ()  [unwired: 2 in, 2 out]
            n165 = property on="Motor" class="Clust (strict)"("Visible"=FALSE) -> ()  [unwired: 2 in, 2 out]
            n166 = property on="Rev/Fwd" class="Clust (strict)"("Visible"=FALSE) -> ()  [unwired: 2 in, 2 out]
            n167 = case shown="\"White Balance  **\"" w299 {
              tunnel: w298 -> [w305 w314 w323 w332 w341 _ w347]
              tunnel: w297 -> [w303 w311 w320 w329 w338 _ _]
              frame "Size  **" {
                n168 = Index Array(array=w303) -> (element=w302:cluster{string[]})  [unwired: 1 in]
                n169 = call <vilib>:"NT Read String.vi"("Name"=w305) -> ("String"=w304:string)  [unwired: 9 in, 1 out]
                n170 = Unbundle(w302) -> (w300:string[])
                n171 = Match First String(2:w300, 3:w304) -> (0:w301:i32)  [unwired: 1 out]
                n172 = property on="Test Ring" class="Ring (strict)"("Value"=w301, "Strings []"=w300) -> ()  [unwired: 2 in, 2 out]
                n173 = property on="Test Ring" class="Ring (strict)"("Visible"=TRUE) -> ()  [unwired: 2 in, 2 out]
                n174 = property on="Test Slider" class="Slide (strict)"("Visible"=FALSE) -> ()  [unwired: 2 in, 2 out]
              }
              frame "White Balance  **" {
                n175 = Index Array(array=w311, index=1) -> (element=w312:cluster{string[]})
                n176 = call <vilib>:"NT Read String.vi"("Name"=w314) -> ("String"=w313:string)  [unwired: 9 in, 1 out]
                n177 = Unbundle(w312) -> (w309:string[])
                n178 = Match First String(2:w309, 3:w313) -> (0:w308:i32)  [unwired: 1 out]
                n179 = property on="Test Ring" class="Ring (strict)"("Value"=w308, "Strings []"=w309) -> ()  [unwired: 2 in, 2 out]
                n180 = property on="Test Ring" class="Ring (strict)"("Visible"=TRUE) -> ()  [unwired: 2 in, 2 out]
                n181 = property on="Test Slider" class="Slide (strict)"("Visible"=FALSE) -> ()  [unwired: 2 in, 2 out]
              }
              frame "Exposure  **" {
                n182 = Index Array(array=w320, index=2) -> (element=w321:cluster{string[]})
                n183 = call <vilib>:"NT Read String.vi"("Name"=w323) -> ("String"=w322:string)  [unwired: 9 in, 1 out]
                n184 = Unbundle(w321) -> (w317:string[])
                n185 = Match First String(2:w317, 3:w322) -> (0:w318:i32)  [unwired: 1 out]
                n186 = property on="Test Ring" class="Ring (strict)"("Value"=w318, "Strings []"=w317) -> ()  [unwired: 2 in, 2 out]
                n187 = property on="Test Ring" class="Ring (strict)"("Visible"=TRUE) -> ()  [unwired: 2 in, 2 out]
                n188 = property on="Test Slider" class="Slide (strict)"("Visible"=FALSE) -> ()  [unwired: 2 in, 2 out]
              }
              frame "Exposure Priority  **" {
                n189 = Index Array(array=w329, index=3) -> (element=w330:cluster{string[]})
                n190 = call <vilib>:"NT Read String.vi"("Name"=w332) -> ("String"=w331:string)  [unwired: 9 in, 1 out]
                n191 = Unbundle(w330) -> (w326:string[])
                n192 = Match First String(2:w326, 3:w331) -> (0:w327:i32)  [unwired: 1 out]
                n193 = property on="Test Ring" class="Ring (strict)"("Value"=w327, "Strings []"=w326) -> ()  [unwired: 2 in, 2 out]
                n194 = property on="Test Ring" class="Ring (strict)"("Visible"=TRUE) -> ()  [unwired: 2 in, 2 out]
                n195 = property on="Test Slider" class="Slide (strict)"("Visible"=FALSE) -> ()  [unwired: 2 in, 2 out]
              }
              frame "Color Enable  **" {
                n196 = Index Array(array=w338, index=4) -> (element=w339:cluster{string[]})
                n197 = call <vilib>:"NT Read String.vi"("Name"=w341) -> ("String"=w340:string)  [unwired: 9 in, 1 out]
                n198 = Unbundle(w339) -> (w335:string[])
                n199 = Match First String(2:w335, 3:w340) -> (0:w336:i32)  [unwired: 1 out]
                n200 = property on="Test Ring" class="Ring (strict)"("Value"=w336, "Strings []"=w335) -> ()  [unwired: 2 in, 2 out]
                n201 = property on="Test Ring" class="Ring (strict)"("Visible"=TRUE) -> ()  [unwired: 2 in, 2 out]
                n202 = property on="Test Slider" class="Slide (strict)"("Visible"=FALSE) -> ()  [unwired: 2 in, 2 out]
              }
              frame Default {
                n203 = property on="Test Ring" class="Ring (strict)"("Visible"=FALSE) -> ()  [unwired: 2 in, 2 out]
                n204 = property on="Test Slider" class="Slide (strict)"("Visible"=FALSE) -> ()  [unwired: 2 in, 2 out]
              }
              frame "Brightness  **", "Color Level  **", "Compression  **", "FPS  **", "Sharpness  **" {
                n205 = call <vilib>:"NT Read Number.vi"("Name"=w347) -> ("Numeric"=w346:dbl)  [unwired: 9 in, 1 out]
                n206 = local write "Test Slider"(w346) -> ()
                n207 = property on="Test Slider" class="Slide (strict)"("Visible"=TRUE, "Scale.Maximum"=100.0 ("Scale.Range:Maximum")) -> ()  [unwired: 2 in, 2 out]
                n208 = property on="Test Ring" class="Ring (strict)"("Visible"=FALSE) -> ()  [unwired: 2 in, 2 out]
              }
            }
          }
        }
        n209 = property on="Progress" class="Clust (strict)"("Visible"=FALSE) -> ()  [unwired: 2 in, 2 out]
      }
      event "Test Name": Mouse Enter {
        # "Populate the ring with the list of tests"
        n210 = event-data() -> ()  [unwired: 1 in, 1 out]
        n211 = call <vilib>:"NT Read String Array.vi"("Name"="/TestMode/TestList") -> ("String Array"=w355:string[])  [unwired: 9 in, 1 out]
        n212 = Build Array (concatenate)("Select the test to run...", w355) -> (w354:string[])
        n213 = property on="Test Name" class="Ring (strict)"("Strings []"=w354) -> ()  [unwired: 2 in, 2 out]
      }
      event "Test Name": Value Change {
        w357 = FALSE ("Visible")
        # "Tell the robot the test name to run"
        n214 = event-data() -> ("NewVal"=w361:u16)  [unwired: 1 in]
        n215 = property on="Test Name" class="Ring (strict)"() -> ("Strings []"=w362:string[])  [unwired: 2 in, 2 out]
        n216 = local write "Progress"(T8 {"Test Progress"=0, "Test Progress Text"=""} ("Progress")) -> ()
        n217 = Index Array(array=w362, index=w361) -> (element=w360:string)
        n218 = call <vilib>:"NT Write String.vi"("String"=w360, "Name"="/TestMode/TestName") -> ()  [unwired: 9 in, 1 out]
        n219 = property on="Progress" class="Clust (strict)"("Visible"=TRUE) -> ()  [unwired: 2 in, 2 out]
        n220 = property on="Motor" class="Clust (strict)"("Visible"=w357) -> ()  [unwired: 2 in, 2 out]
        n221 = property on="Test Slider" class="Slide (strict)"("Visible"=w357) -> ()  [unwired: 2 in, 2 out]
        n222 = property on="On/Off" class="Bool (strict)"("Visible"=w357) -> ()  [unwired: 2 in, 2 out]
        n223 = property on="Rev/Fwd" class="Clust (strict)"("Visible"=w357) -> ()  [unwired: 2 in, 2 out]
        n224 = property on="Test Ring" class="Ring (strict)"("Visible"=w357) -> ()  [unwired: 2 in, 2 out]
      }
      event Mouse Enter {
        # "Populate the combo box with the list of autonomous options"
        n225 = event-data() -> ()  [unwired: 1 in, 1 out]
        n226 = call <vilib>:"NT Read String Array.vi"("Name"="Auto List") -> ("String Array"=w364:string[])  [unwired: 9 in, 1 out]
        n227 = property on="Select Auto" class="CmbBox (strict)"("Strings[]"=w364) -> ()  [unwired: 2 in, 2 out]
      }
      event Value Change {
        # "User modified the Auto Selection. Write to NT variable so robot knows."
        n228 = event-data() -> ("NewVal"=w367:T3)  [unwired: 1 in]
        n229 = call <vilib>:"NT Write String.vi"("String"=w367, "Name"="Auto Selector") -> ()  [unwired: 9 in, 1 out]
      }
      event "Command Selection": Value Change {
        # "Get the params and show in table"
        n230 = event-data() -> ("NewVal"=w373:i32)  [unwired: 1 in]
        n231 = property on="Command Selection" class="MCListbox (strict)"() -> ("ItemNames"=w371:string[][])  [unwired: 2 in, 2 out]
        n232 = call <vilib>:"WPI_DashboardUpdate Command Params.vi"("NewVal"=w373, "Commands"=w371, "Param Tbl"=w372) -> ()  [unwired: 8 in, 1 out]
      }
      event "Execute Command": Value Change {
        # "Started one, Unique ID holds\nresponse"
        n233 = event-data() -> ()  [unwired: 1 in, 1 out]
        n234 = property on="Command Selection" class="MCListbox (strict)"() -> ("ItemNames"=w384:string[][])  [unwired: 2 in, 2 out]
        n235 = Index Array(array=w384, index (row)="Command Selection", index (col)=0) -> (element=w382:string)
        n236 = call <vilib>:"Invoke Commands.vi"("Command Params"="Command Params", "Function Name"=w382) -> ("Params"=w378:u8, "Started"=w377:bool)  [unwired: 7 in, 1 out]
        n237 = Array Subset(array="Command Params", length (row)=w378) -> (w379:string[][])  [unwired: 3 in]
        n238 = Select(t="Executing" ("Cmd Status"), s=w377, f="" ("Cmd Status")) -> (s? t:f=→"Cmd Status":string)
      }
      event "Command Selection": Double Click {
        n239 = event-data() -> ("Row"=w392:i32)  [unwired: 1 in]
        n240 = property on="Command Selection" class="MCListbox (strict)"() -> ("ItemNames"=w395:string[][])  [unwired: 2 in, 2 out]
        n241 = local read "Command Params"() -> (w391:string[][])
        n242 = Index Array(array=w395, index (row)=w392, index (col)=0) -> (element=w393:string)
        n243 = call <vilib>:"Invoke Commands.vi"("Command Params"=w391, "Function Name"=w393) -> ("Params"=w390:u8, "Started"=w385:bool)  [unwired: 7 in, 1 out]
        n244 = Array Subset(array=w391, length (row)=w390) -> (w389:string[][])  [unwired: 3 in]
        n245 = Select(t="Executing" ("Cmd Status"), s=w385, f="" ("Cmd Status")) -> (s? t:f=w386:string)
        n246 = local write "Cmd Status"(w386) -> ()
      }
      event "CheckList": Double Click {
        # "Shift clears all"
        # "Update symbols on the listbox"
        n247 = event-data() -> ("PlatMods.Shift"=w397:bool, "Row"=w399:i32)  [unwired: 1 in]
        n248 = case shown="True" w397 {
          tunnel: w399 -> [w403 _]
          tunnel: 1 -> [w402 _]
          frame False {
            n249 = property on="CheckList" class="LstBox (strict)"() -> ("Item Symbols"=w401:i32[])  [unwired: 2 in, 2 out]
            n250 = Replace Array Subset(array=w401, new element=w402, index=w403) -> (w400:i32[])
            n251 = property on="CheckList" class="LstBox (strict)"("Item Symbols"=w400) -> ()  [unwired: 2 in, 2 out]
          }
          frame True {
            w404 = 0 ("Top Row")
            n252 = property on="CheckList" class="LstBox (strict)"() -> ("Number of Rows"=w406:u32)  [unwired: 2 in, 2 out]
            n253 = Initialize Array(0, w406) -> (w405:i32[])
            n254 = property on="CheckList" class="LstBox (strict)"("Top Row"=w404, "Value"=w404, "Item Symbols"=w405) -> ()  [unwired: 2 in, 2 out]
          }
        }
      }
      event "CheckList": Key Down {
        # "Update symbols on the listbox\nLeft and right keys check and uncheck"
        n255 = event-data() -> ("VKey"=w410:T21)  [unwired: 1 in]
        n256 = case shown="\"Left\", \"Right\"" w410 {
          selector: w410 -> [w415 _]
          tunnel: eventvkey."Left" ("VKey") -> [w413 _]
          frame "Left", "Right" {
            n257 = Equal?(x=w413, y=w415) -> (x = y?=w414:bool)
            n258 = Select(t=0, s=w414, f=1) -> (s? t:f=w416:i32)
            n259 = property on="CheckList" class="LstBox (strict)"() -> ("Item Symbols"=w419:i32[])  [unwired: 2 in, 2 out]
            n260 = Replace Array Subset(array=w419, new element=w416, index="CheckList") -> (w418:i32[])
            n261 = property on="CheckList" class="LstBox (strict)"("Item Symbols"=w418) -> ()  [unwired: 2 in, 2 out]
          }
          frame Default {
          }
        }
      }
      event "Motor.Enable": Value Change {
        # "When the test mode otor enable helper is set, update that\ntree row item's value"
        n262 = event-data() -> ("NewVal"=w425:bool)  [unwired: 1 in]
        n263 = Unbundle("Motor") -> ("Value"=w424:dbl)  [unwired: 1 out]
        n264 = Select(t=w424, s=w425, f=0.0) -> (s? t:f=w422:dbl)
        n265 = call <vilib>:"NT Write Number.vi"("Numeric"=w422, "Name"=w421) -> ()  [unwired: 9 in, 1 out]
      }
      event "Test Slider": Value Change {
        # "When the test mode slider helper is set, update that\ntree row item's value"
        n266 = event-data() -> ("NewVal"=w428:dbl)  [unwired: 1 in]
        n267 = call <vilib>:"NT Write Number.vi"("Numeric"=w428, "Name"=w429) -> ()  [unwired: 9 in, 1 out]
      }
      event "On/Off": Value Change {
        # "When the test mode on/off helper value is set, update that\ntree row item's value"
        n268 = event-data() -> ("NewVal"=w433:bool)  [unwired: 1 in]
        n269 = Boolean To (0,1)(Boolean=w433) -> (0, 1=w432:i16)
        n270 = call <vilib>:"NT Write Number.vi"("Numeric"=w432, "Name"=w431) -> ()  [unwired: 9 in, 1 out]
      }
      event "Rev/Fwd": Value Change {
        # "When the test mode helper value for relays is set, update that\ntree row item's value"
        n271 = event-data() -> ("NewVal.Forward"=w441:bool, "NewVal.Reverse"=w440:bool)  [unwired: 1 in]
        n272 = Boolean To (0,1)(Boolean=w441) -> (0, 1=w437:i16)
        n273 = Boolean To (0,1)(Boolean=w440) -> (0, 1=w439:i16)
        n274 = Negate(x=w439) -> (-x=w438:i16)
        n275 = Add(x=w437, y=w438) -> (x+y=w436:i16)
        n276 = call <vilib>:"NT Write Number.vi"("Numeric"=w436, "Name"=w435) -> ()  [unwired: 9 in, 1 out]
      }
      event "Test Ring": Value Change {
        # "When a test mode helper value is selected from the ring,\nset the tree item's variable to the string value"
        n277 = event-data() -> ("NewVal"=w445:u16)  [unwired: 1 in]
        n278 = property on="Test Ring" class="Ring (strict)"() -> ("Strings []"=w446:string[])  [unwired: 2 in, 2 out]
        n279 = Index Array(array=w446, index=w445) -> (element=w444:string)
        n280 = call <vilib>:"NT Write String.vi"("String"=w444, "Name"=w443) -> ()  [unwired: 9 in, 1 out]
      }
      event "Rec Mode": Value Change {
        # "Update globals for recording mode and path to read log from.\nClear when logging and let NetworkTables set path for vision to\nuse."
        n281 = event-data() -> ("NewVal"=w457:enum32{"Stop", "Record", "Playback"})  [unwired: 1 in]
        n282 = global write "WPI_DashboardLogging Global.vi" "Logging Filename"(path "") -> ()
        n283 = global write "WPI_DashboardLogging Global.vi" "Recording"(w457) -> ()
        n284 = case shown="\"Playback\"" w457 {
          tunnel: w456 -> [_ w459 w468]
          tunnel: [_ _ w467] -> w454
          tunnel: [_ _ w466] -> _
          tunnel: w452 -> [_ _ w464]
          tunnel: cluster{i32, i32} {-250, 170} -> [_ _ w463]
          tunnel: [_ _ T22 {"Image Size"=TRUE, "Image Type"=TRUE, "Pixel Value"=TRUE, "ROI Information"=TRUE, "Zoom Factor"=FALSE} ("Image Information Shown:All Elements")] -> w450
          tunnel: [_ _ TRUE ("Zoom Factor")] -> w449
          tunnel: w448 -> [_ _ w460]
          frame Default {
          }
          frame "Stop", "Record" {
            # "Place Window too"
            n285 = invoke class="VI" method="FP.Close"(reference=w459) -> (reference out=w458:refnum<vi>)  [unwired: 2 in, 2 out]
            n286 = invoke class="VI" method="Abort VI"(reference=w458) -> ()  [unwired: 2 in, 3 out]
          }
          frame "Playback" {
            n287 = call "Open Playback Panel.vi"("Offset"=w463, "DB VI Ref"=w464, "Playback in"=w468) -> ("Playback out"=w465:refnum<vi>)  [unwired: 8 in]
            n288 = register-events(w465, w460) -> (reference out=w467:refnum<event-registration>, error out=w466:errorcluster)  [unwired: 2 in]
          }
        }
        n289 = property on="Camera Image" class="ImageControl"("Image Information Shown"=w450, "Image Information Visible"=w449) -> ()  [unwired: 2 in, 2 out]
        n290 = call <vilib>:"WPI_DashboardNT Log FieldName Cache.vi"("Operation"=enum16{"Lookup/Add", "Index", "Clear"}."Clear") -> ()  [unwired: 8 in, 3 out]
      }
      event Panel Close {
        w470 = enum32{"Stop", "Record", "Playback"}."Stop" ("Rec Mode")
        # "Playback window has been closed, abort"
        n291 = event-data() -> ()  [unwired: 1 in, 4 out]
        n292 = local write "Rec Mode"(w470) -> ()
        n293 = global write "WPI_DashboardLogging Global.vi" "Recording"(w470) -> ()
      }
      event Panel Close {
        # "Abort playback window and ourself"
        n294 = event-data() -> ()  [unwired: 1 in, 4 out]
        n295 = invoke class="VI" method="FP.Close"(reference=w474) -> (reference out=w473:refnum<vi>)  [unwired: 2 in, 2 out]
        n296 = invoke class="VI" method="Abort VI"(reference=w473) -> (error out=w472:errorcluster)  [unwired: 2 in, 2 out]
        n297 = invoke class="VI" method="Abort VI"(error in=w472) -> ()  [unwired: 2 in, 3 out]
      }
      event User Event {
        n298 = event-data() -> ("IDs"=w481:cluster{"RPC field ID":u16, "Unique ID":u16}, "String"=w480:string)  [unwired: 1 in]
        n299 = Bundle("IDs"=w481, "String"=w480) -> (w479:T10)  [unwired: 1 in]
        n300 = call <vilib>:"Retrieve RPC Response.vi"("RPC Response"=w479) -> ("Output"=w477:string[][])  [unwired: 10 in]
        n301 = Build Array (concatenate)(w475, w477) -> (w476:string[][])
        n302 = local write "Command Params"(w476) -> ()
        n303 = local write "Cmd Status"("" ("Cmd Status")) -> ()
      }
      event "Tree": Double Click {
        n304 = event-data() -> ("PlatMods"=w485:T25, "Tag"=w484:string)  [unwired: 1 in]
        n305 = Unbundle(w485) -> ("Shift"=w483:bool)  [unwired: 4 out]
        n306 = Not(x=w483) -> (.not. x?=w482:bool)
        n307 = call <vilib>:"NT Update Persistence.vi"("Persistence"=w482, "Name"=w484) -> ()  [unwired: 9 in, 1 out]
      }
    }
  }
  n308 = while {
    tunnel: w80 -> [w488]
    i -> [w491]
    stop <- FALSE stop-if-true
    n309 = Wait (ms)(milliseconds to wait=u32 100) -> ()  [unwired: 1 out]
    n310 = case shown="\"Playback\"" "Rec Mode" {
      tunnel: w491 -> [_ _ w506]
      tunnel: [u32 2829099 ("Base Color") u32 11141120 ("Target Color") w495] -> w487
      frame "Stop", Default {
        # "Reset the color, extra updates don't cost much"
      }
      frame "Record" {
      }
      frame "Playback" {
        # "Playback"
        n311 = Quotient & Remainder(x=w506, y=u32 50 ("milliseconds to wait")) -> (x-y*floor(x/y)=w502:u32)  [unwired: 1 out]
        n312 = Divide(x=w502, y=u32 50 ("milliseconds to wait")) -> (x/y=w499:dbl)
        n313 = Multiply(x=6.283185307179586, y=w499) -> (x*y=w504:dbl)
        n314 = Sine(x=w504) -> (sin(x)=w503:dbl)
        n315 = Absolute Value(x=w503) -> (abs(x)=w496:dbl)
        n316 = call "Interpolate RGB Color.vi"("Proportion"=w496, "Target Color"=u32 30976, "Base Color"=u32 2829099) -> ("Result Color"=w495:u32)  [unwired: 8 in]
      }
    }
    n317 = property class="Pane"(reference=w488, "PaneColor"=w487) -> ()  [unwired: 1 in, 2 out]
  }
  n318 = local write "Dashboard Tab"(T2."Drive" ("Dashboard Tab")) -> ()
  n319 = property on="On/Off" class="Bool (strict)"("Visible"=w49) -> ()  [unwired: 2 in, 2 out]
  n320 = property on="Motor" class="Clust (strict)"("Visible"=w49) -> ()  [unwired: 2 in, 2 out]
  n321 = property on="Progress" class="Clust (strict)"("Visible"=w49) -> ()  [unwired: 2 in, 2 out]
  n322 = property on="Test Ring" class="Ring (strict)"("Visible"=w49) -> ()  [unwired: 2 in, 2 out]
  n323 = property on="Rev/Fwd" class="Clust (strict)"("Visible"=w49) -> ()  [unwired: 2 in, 2 out]
  n324 = while {
    tunnel: u16 1741 ("timeout ms (25000)") -> [w508]
    stop <- FALSE stop-if-true
    n325 = TCP Create Listener(10:w508) -> (0:w507:errorcluster, 3:w509:refnum<k5>)  [unwired: 4 in, 1 out]
    n326 = case shown="No Error" w507 {
      selector: w507 -> [w511 _]
      tunnel: w509 -> [w512 _]
      frame No Error {
        n327 = while {
          tunnel: w512 -> [w515]
          tunnel: w511 -> [w514]
          stop <- FALSE stop-if-true
          n328 = TCP Wait On Listener(8:w514, 11:w515) -> (0:w516:errorcluster, 4:w517:refnum<k5>)  [unwired: 2 in, 3 out]
          n329 = local write "TCP"(w517) -> ()
          n330 = case shown="No Error" w516 {
            frame No Error {
            }
            frame Error {
              n331 = Wait (ms)(milliseconds to wait=u32 1000) -> ()  [unwired: 1 out]
            }
          }
        }
      }
      frame Error {
        n332 = Wait (ms)(milliseconds to wait=u32 1000) -> ()  [unwired: 1 out]
      }
    }
  }
  n333 = local write "Command Selection"(u16 0 ("milliseconds to wait")) -> ()
  n334 = local write "Command Params"(string[][] [] ("Command Params")) -> ()
  n335 = global write "WPI_DashboardLogging Global.vi" "Recording"(w74) -> ()
  n336 = local write "Rec Mode"(w74) -> ()
  n337 = call <vilib>:"NT Write String.vi"("String"="Select Auto", "Name"="Auto Selector") -> ()  [unwired: 9 in, 1 out]
  n338 = property on="Control Select" class="Enum (strict)"() -> ("Strings []"=w3:string[], "Value"=w1:T6)  [unwired: 2 in, 2 out]
  n339 = Index Array(array=w3, index=w1) -> (element=w2:string)
  n340 = call <vilib>:"NT Write String.vi"("String"=w2, "Name"="Control Selector") -> ()  [unwired: 9 in, 1 out]
  n341 = Build Array("Left", "Right", "Distance") -> (w14:dbl[])
  n342 = call-poly <vilib>:"NT Write Value.vi"("Boolean"="Toggle LED", "Name"="Toggle Backlight") -> ()  [unwired: 9 in, 1 out]
  n343 = call-poly <vilib>:"NT Write Value.vi"("Numeric Array"=w14, "Name"="Drive to Distance Tester") -> ()  [unwired: 9 in, 1 out]
  n344 = call-poly <vilib>:"NT Write Value.vi"("Boolean"="Nintendo Camera Switch", "Name"="Nintendo Camera Switch") -> ()  [unwired: 9 in, 1 out]
